vi "Temperature Limit.vi"() -> ()   [LabVIEW 2015]
doc: "This VI simulates the acquisition of temperature, graphs the temperature, and notifies the user if the temperature is over the limit."
panel:
  in  "Start":bool
  in  "Delta t (ms)":i32(slide)=400 scale=50.0..500.0
  in  "Stop":bool
  in  "High Limit":dbl=28.0 format="%.2f"
  out "Temperature":cluster{"Temperature":dbl, "High Limit":dbl}(graph)={"Temperature"=85.88749999999999, "High Limit"=80.0}
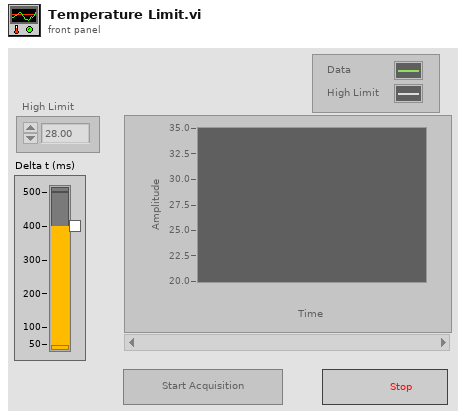
[diagram p1: front panel]
types:
  T1 = enum8{"Enabled", "Disabled", "Disabled and Grayed Out"}
  T2 = enum16{"Always On", "Always Off", "Off While Running"}
  T3 = cluster{"Temperature Value":dbl, "High Limit":dbl}
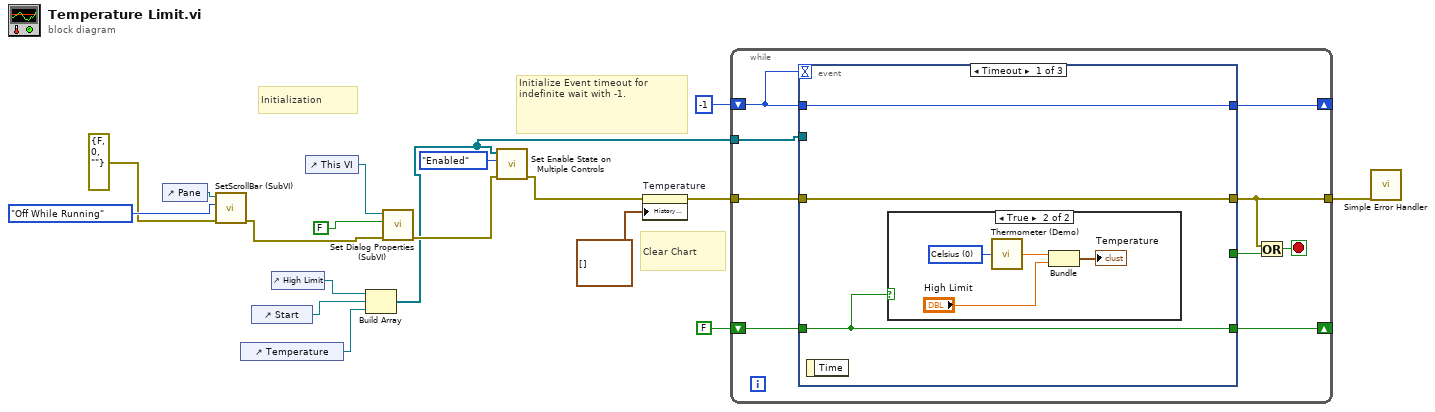
[diagram p0: block diagram]
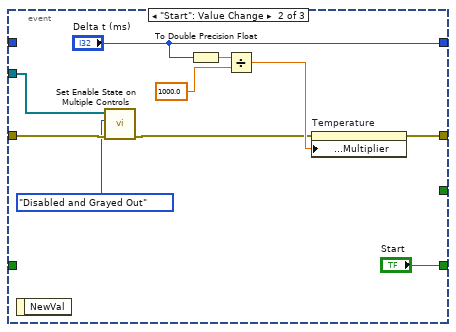
[diagram p3: hidden frame]
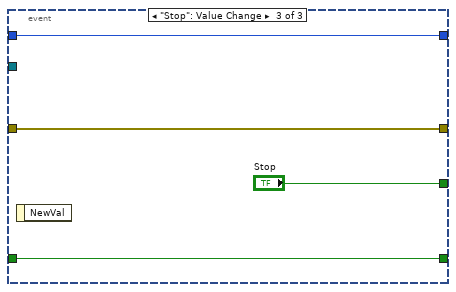
[diagram p4: hidden frame]
diagram:
  # "Clear Chart"
  # "Initialize Event timeout for indefinite wait with -1."
  # "Initialization"
  n1 = control-ref of="Pane"() -> (w8:refnum<vi>)
  n2 = call "SetScrollBar (SubVI).vi"("error in (no error)"=errorcluster {"status"=FALSE, "code"=0, "source"=""}, "Horizontal Scrollbar Visibility"=T2."Off While Running", "Pane in"=w8) -> ("error out"=w11:errorcluster)  [unwired: 7 in, 1 out]
  n3 = control-ref of="Temperature"() -> (w6:refnum<vi>)
  n4 = control-ref of="Start"() -> (w1:refnum<vi>)
  n5 = control-ref of="High Limit"() -> (w7:refnum<vi>)
  n6 = control-ref of="This VI"() -> (w12:refnum<vi>)
  n7 = Build Array(w7, w1, w6) -> (w2:refnum<vi>[])
  n8 = call "Set Dialog Properties (SubVI).vi"("error in (no error)"=w11, "Boolean"=FALSE, "VI in"=w12) -> ("error out"=w4:errorcluster)  [unwired: 7 in, 1 out]
  n9 = call "Set Enable State on Multiple Controls.vi"("Error In"=w4, "Disabled State"=T1."Enabled", "Controls"=w2) -> ("Error Out"=w5:errorcluster)  [unwired: 8 in]
  n10 = property on="Temperature" class="WFChart (strict)"(error in=w5, "History Data"=cluster{"Temperature":dbl, "High Limit":dbl}[] []) -> (error out=w17:errorcluster)  [unwired: 1 in, 1 out]
  n11 = while {
    tunnel: w17 -> [w27]
    tunnel: [w25] -> w15
    shift-right: [w23] -> _
    shift-left: FALSE ("Start") -> [w22]
    shift-right: [w21] -> _
    shift-left: -1 ("Delta t (ms)") -> [w20]
    tunnel: w2 -> [w19]
    stop <- w26 stop-if-true
    n12 = event shown="[0] Timeout" {
      selector: _ -> [_ _ _]
      dyn-events: _ -> [_ _ _]
      timeout: w20 -> [_ _ _]
      tunnel: [_ _ "Stop"] -> w24
      tunnel: w27 -> [w30 w38 w47]
      tunnel: [w30 w44 w47] -> w25
      tunnel: [w28 "Start" w46] -> w23
      tunnel: w22 -> [w28 _ w46]
      tunnel: [w29 "Delta t (ms)" w45] -> w21
      tunnel: w20 -> [w29 _ w45]
      tunnel: w19 -> [_ w36 _]
      event Timeout {
        n13 = event-data() -> ()  [unwired: 1 in, 1 out]
        n14 = case shown="True" w28 {
          frame False {
          }
          frame True {
            w31 = u16 0 items=["Celsius", "Fahrenheit"] ("Units (0: Celsius)")
            n15 = call "Thermometer (Demo).vi"("Units (0: Celsius)"=w31) -> ("Temperature Value"=w32:dbl)
            n16 = Bundle("Temperature Value"=w32, "High Limit"="High Limit") -> (→"Temperature":T3)  [unwired: 1 in]
          }
        }
      }
      event "Start": Value Change {
        n17 = event-data() -> ()  [unwired: 1 in, 1 out]
        n18 = call "Set Enable State on Multiple Controls.vi"("Error In"=w38, "Disabled State"=T1."Disabled and Grayed Out", "Controls"=w36) -> ("Error Out"=w37:errorcluster)  [unwired: 8 in]
        n19 = To Double Precision Float(number="Delta t (ms)") -> (double precision float=w43:dbl)
        n20 = Divide(x=w43, y=1000.0) -> (x/y=w41:dbl)
        n21 = property on="Temperature" class="WFChart (strict)"(error in=w37, "X Scale.Offset and Multiplier:Multiplier"=w41) -> (error out=w44:errorcluster)  [unwired: 1 in, 1 out]
      }
      event "Stop": Value Change {
        n22 = event-data() -> ()  [unwired: 1 in, 1 out]
      }
    }
    n23 = Or(x=w25, y=w24) -> (x .or. y?=w26:bool)
  }
  n24 = call <vilib>:"Simple Error Handler.vi"("error in (no error)"=w15) -> ()  [unwired: 4 in, 5 out]
